vi "DiJian_mess.vi"(7 "Timeout(默认:5ms)":i32=5, 8 "error in":errorcluster, 9 "COM通道":u32=1, 10 "索引":i32, 11 "VISA资源名称":refnum<visa-resource-name>) -> (0 "error out 2":errorcluster, 1 "timeout":bool, 3 "VISAout":refnum<visa-resource-name>)   [LabVIEW 2012]
uses:
  <vilib>/GPower/VIRegister/Library/SubVIs/FindRegisterData.vi
  <vilib>/GPower/VIRegister/Library/SubVIs/ReadSub.vi
  <vilib>/GPower/VIRegister/Library/QManager/GetRegisterData.vi
  <vilib>/GPower/Error/Library/SetError.vi
  <vilib>/GPower/Error/Library/FilterCodes.vi
  <vilib>/GPower/Error/Library/Filter/FilterMulti.vi
  <vilib>/GPower/VIRegister/Library/QManager/QManagerAction.vi
  <vilib>/GPower/Error/Library/ErrorType.vi
  <vilib>/GPower/Error/Library/SplitAppended.vi
  <vilib>/GPower/Error/Library/SubVIs/ExplanationToError.vi
  <vilib>/GPower/VIRegister/Library/QManager/GetQName.vi
  <vilib>/GPower/VIRegister/Library/QManager/StartQManager.vi
  <vilib>/Utility/error.llb/Trim Whitespace.vi
  <vilib>/dlg_ctls.llb/Space Constant.vi
  <vilib>/Utility/error.llb/Error Code Database.vi
  <vilib>/GPower/Error/Library/SubVIs/SetStatus.vi
  <vilib>/GPower/Error/Library/AppendErrors.vi
  <vilib>/GPower/Error/Library/Append/AppendSingle.vi
  com/TONGXUN/write32.vi
  com/TONGXUN/write8.vi
  <vilib>/GPower/VIRegister/VIRegister.lvlib
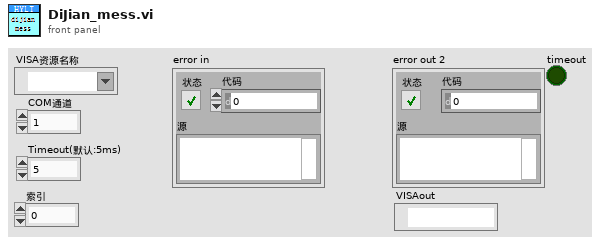
[diagram p1: front panel]
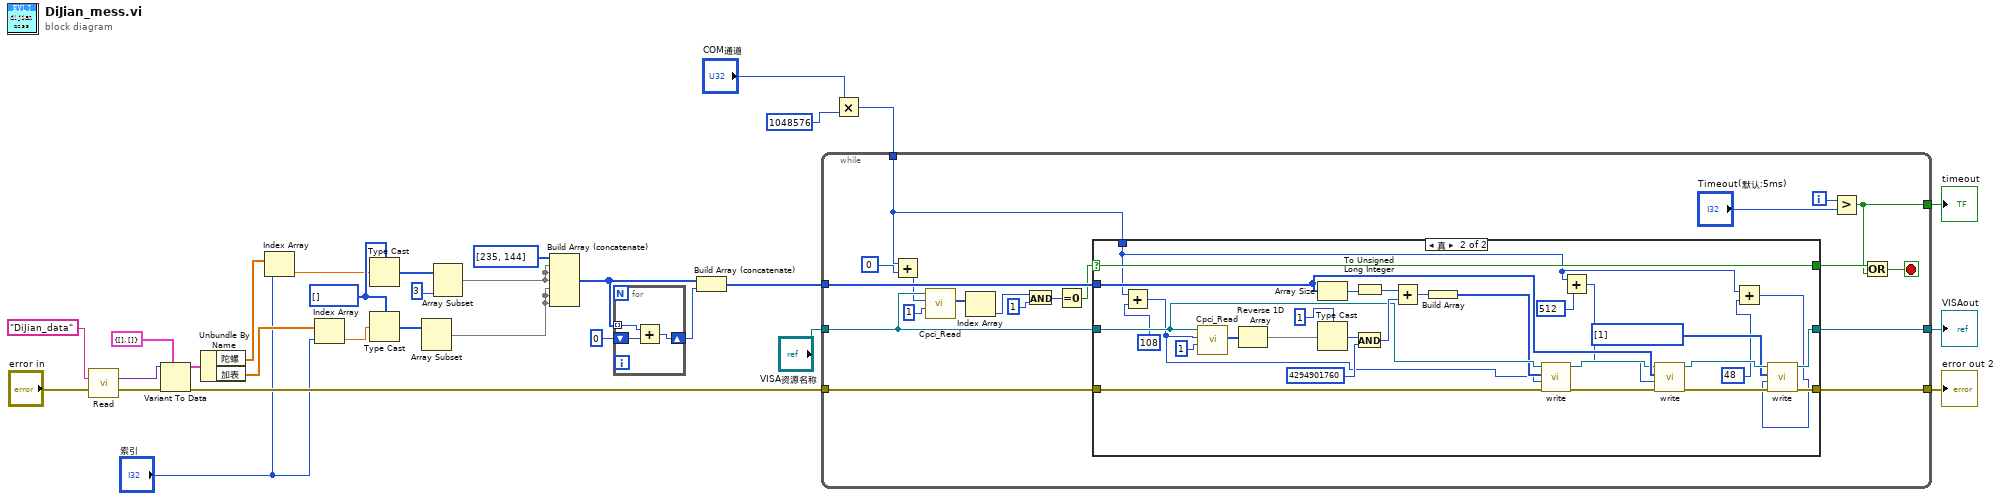
[diagram p0: block diagram]
diagram:
  w26 = u8[] []
  n1 = call <vilib>:"Read.vi"("Register name"="DiJian_data", "Error in"="error in") -> ("Register value"=w17:variant, "Error out"=w8:errorcluster)  [unwired: 10 in, 2 out]
  n2 = Variant To Data(error in=w8, type=cluster{"陀螺":dbl[], "加表":dbl[]} {"陀螺"=[], "加表"=[]} ("输入簇"), Variant=w17) -> (data=w18:cluster{"陀螺":dbl[], "加表":dbl[]}, error out=w7:errorcluster)
  n3 = Unbundle By Name(w18) -> ("陀螺"=w19:dbl[], "加表"=w20:dbl[])
  n4 = Index Array(array=w19, index="索引") -> (element=w21:dbl)
  n5 = Index Array(array=w20, index="索引") -> (element=w25:dbl)
  n6 = Type Cast(type=w26, x=w21) -> (*(type *) &x=w22:u8[])
  n7 = Type Cast(type=w26, x=w25) -> (*(type *) &x=w24:u8[])
  n8 = Array Subset(array=w24) -> (w14:u8[])  [unwired: 2 in]
  n9 = Array Subset(array=w22, length=3 ("长度")) -> (w15:u8[])  [unwired: 1 in]
  n10 = Build Array (concatenate)(u8[] [235, 144] ("数组"), w15, w15, w15, w14, w14, w14) -> (w10:u8[])
  n11 = for {
    tunnel: w10 -> [w33] mode=indexing
    shift-right: [w31] -> w11
    shift-left: u8 0 ("y") -> [w32]
    n12 = Add(x=w33, y=w32) -> (x+y=w31:u8)
  }
  n13 = Build Array (concatenate)(w10, w11) -> (w9:u8[])
  n14 = Multiply(x="COM通道", y=u32 1048576 ("基地址")) -> (x*y=w3:u32)
  n15 = while {
    tunnel: "VISA资源名称" -> [w49]
    tunnel: w9 -> [w52]
    tunnel: w7 -> [w51]
    tunnel: [w50] -> w29
    tunnel: [w38] -> w28
    tunnel: [w37] -> w27
    tunnel: w3 -> [w34]
    i -> [w42]
    stop <- w40 stop-if-true
    n16 = Add(x=w34, y=u32 0 ("基地址")) -> (x+y=w35:u32)
    n17 = call "Cpci_Read.vi"("u32_len"=1, "基地址"=w35, "VISA资源名称"=w49) -> ("U8"=w47:u8[])  [unwired: 6 in, 2 out]
    n18 = Index Array(array=w47) -> (element=w46:u8)  [unwired: 1 in]
    n19 = And(x=w46, y=u8 1) -> (x .and. y?=w44:u8)
    n20 = Equal To 0?(x=w44) -> (x = 0?=w43:bool)
    n21 = case shown="真" w43 {
      selector: w43 -> [w55 w77]
      tunnel: w49 -> [w53 w66]
      tunnel: w52 -> [_ w84]
      tunnel: w51 -> [w54 w83]
      tunnel: [w54 w80] -> w50
      tunnel: [w55 w77] -> w39
      tunnel: [w53 w75] -> w37
      tunnel: w34 -> [_ w58]
      frame False {
      }
      frame True {
        n22 = Add(x=w58, y=u32 108 ("偏移量(0)")) -> (x+y=w61:u32)
        n23 = call "Cpci_Read.vi"("u32_len"=1, "基地址"=w61, "VISA资源名称"=w66) -> ("U8"=w70:u8[])  [unwired: 6 in, 2 out]
        n24 = Reverse 1D Array(array=w70) -> (reversed array=w71:u8[])
        n25 = Array Size(array=w84) -> (size(s)=w64:i32)
        n26 = Type Cast(type=u32 1 ("u32_len"), x=w71) -> (*(type *) &x=w73:u32)
        n27 = To Unsigned Long Integer(number=w64) -> (unsigned 32bit integer=w68:u32)
        n28 = And(x=w73, y=u32 4294901760) -> (x .and. y?=w69:u32)
        n29 = Add(x=w68, y=w69) -> (x+y=w67:u32)
        n30 = Build Array(w67) -> (w63:u32[])
        n31 = call-poly "write.vi"("error out"=w83, "起始地址"=w61, "U32"=w63, "VISA资源名称输入"=w66) -> ("error out 2"=w82:errorcluster, "VISA资源名称输出"=w76:refnum<visa-resource-name>)  [unwired: 6 in]
        n32 = Add(x=w58, y=u32 512 ("偏移量(0)")) -> (x+y=w60:u32)
        n33 = call-poly "write.vi"("error out"=w82, "起始地址"=w60, "数组"=w84, "VISA资源名称输入"=w76) -> ("error out 2"=w81:errorcluster, "VISA资源名称 输出"=w79:refnum<visa-resource-name>)  [unwired: 6 in]
        n34 = Add(x=w58, y=u32 48 ("偏移量(0)")) -> (x+y=w56:u32)
        n35 = call-poly "write.vi"("error out"=w81, "起始地址"=w56, "U32"=u32[] [1], "VISA资源名称输入"=w79) -> ("error out 2"=w80:errorcluster, "VISA资源名称输出"=w75:refnum<visa-resource-name>)  [unwired: 6 in]
      }
    }
    n36 = Greater?(x=w42, y="Timeout(默认:5ms)") -> (0:w38:bool)
    n37 = Or(x=w39, y=w38) -> (x .or. y?=w40:bool)
  }
  "error out 2" <- w29
  "timeout" <- w28
  "VISAout" <- w27
